vi "Get Errors After Filtering.vi"(8 "error in (no error)":errorcluster, 11 "Error Manager in":refnum<class "Error Manager.lvclass">) -> (0 "error out":errorcluster, 2 "Array of Errors":T1[](array[typedef]) {"Time Stamp" format="%<%x %.3X>T"}, 3 "Error Manager out":refnum<class "Error Manager.lvclass">)   [LabVIEW 2026, in "TALOS.lvlib" / "Error Manager.lvlib" / "Error Manager.lvclass"]
uses:
  Error Manager.lvclass
  Error Info.ctl
  Error Manager.lvclass/Error Manager.ctl
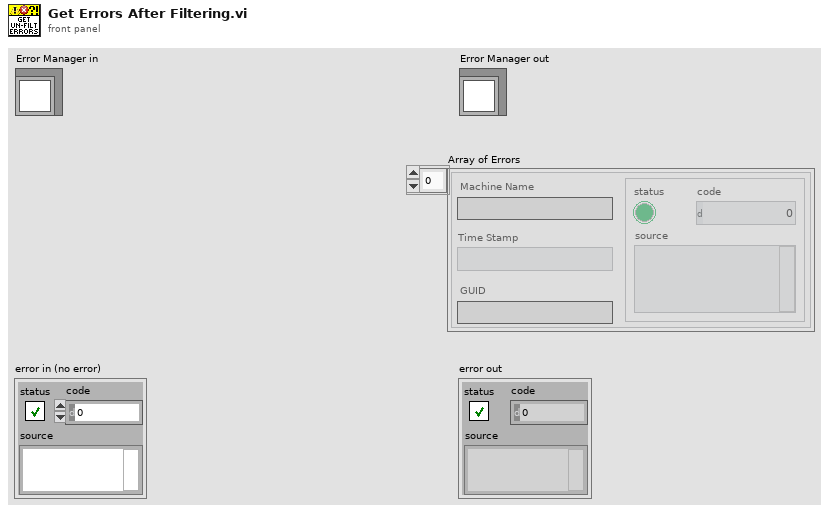
[diagram p1: front panel]
types:
  T1 = typedef "TALOS.lvlib/Error Manager.lvlib/Error Manager.lvclass/Error Info.ctl" = cluster{"error out":errorcluster, "Time Stamp":timestamp, "Machine Name":string, "GUID":string}
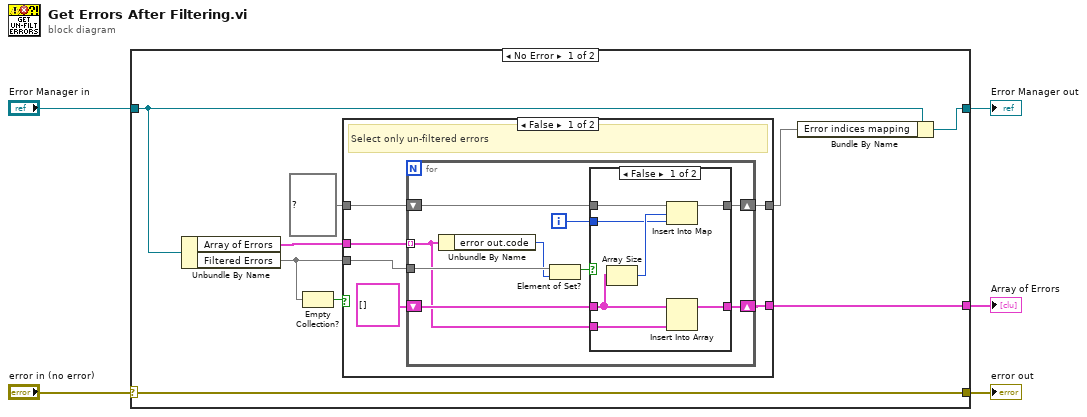
[diagram p0: block diagram]
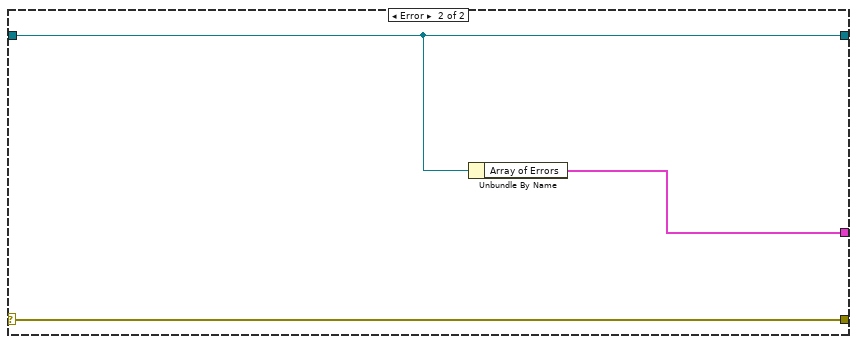
[diagram p4: hidden frame]
diagram:
  n1 = case shown="No Error" "error in (no error)" {
    selector: "error in (no error)" -> [w14 w43]
    tunnel: [w14 w43] -> w4
    tunnel: [w8 w42] -> w2
    tunnel: "Error Manager in" -> [w9 w42]
    tunnel: [w10 w41] -> w1
    frame No Error {
      n2 = Unbundle By Name(w9) -> ("Array of Errors"=w13:T1[], "Filtered Errors"=w11:set{i32})
      n3 = Empty Collection?(1:w11) -> (0:w12:bool)
      n4 = case shown="False" w12 {
        tunnel: w13 -> [w20 w40]
        tunnel: w11 -> [w17 _]
        tunnel: [w18 w40] -> w10
        tunnel: map{i32, i32} {} ("Error indices mapping") -> [w16 w39]
        tunnel: [w15 w39] -> w6
        frame False {
          # "Select only un-filtered errors"
          n5 = for {
            tunnel: w20 -> [w21] mode=indexing
            tunnel: w17 -> [w29]
            shift-right: [w22] -> w18
            shift-left: T1[] [] ("Array") -> [w27]
            shift-right: [w23] -> w15
            shift-left: w16 -> [w24]
            i -> [w25]
            n6 = Unbundle By Name(w21) -> ("error out.code"=w28:i32)
            n7 = Element of Set?(10:w28, 11:w29) -> (3:w26:bool)
            n8 = case shown="False" w26 {
              tunnel: w27 -> [w32 w37]
              tunnel: w25 -> [w30 _]
              tunnel: w24 -> [w35 w38]
              tunnel: [w36 w38] -> w23
              tunnel: [w34 w37] -> w22
              tunnel: w21 -> [w33 _]
              frame False {
                n9 = Array Size(array=w32) -> (size(s)=w31:i32)
                n10 = Insert Into Map(map in=w35, key=w31, value=w30) -> (map out=w36:map{i32, i32})  [unwired: 2 out]
                n11 = Insert Into Array(array=w32, new element=w33) -> (w34:T1[])  [unwired: 1 in]
              }
              frame True {
                # "Filtered error"
              }
            }
          }
        }
        frame True {
          # "Nothing to filter, return all erors"
        }
      }
      n12 = Bundle By Name(cluster=w9, "Error indices mapping"=w6) -> (w8:refnum<class "Error Manager.lvclass">)
    }
    frame Error {
      n13 = Unbundle By Name(w42) -> ("Array of Errors"=w41:T1[])
    }
  }
  "error out" <- w4
  "Error Manager out" <- w2
  "Array of Errors" <- w1
